vi "Calculate Global Grid Points.vi"(9 "steering frame position":T1, 10 "pictures size (units)":cluster{"width":dbl, "height":dbl}, 11 "grid spacing":dbl=1.0) -> (2 "y":dbl[](array[numeric]), 3 "x":dbl[](array[numeric]))   [LabVIEW 2017, in "NI_Robotics_Configure Steering Frame.lvlib"]
uses:
  <vilib>/robotics/Dialog/Configure Steering Frame/NI_Robotics_Configure Steering Frame.lvlib
  <vilib>/Analysis/coordinate.llb/2D Cartesian Coordinate Shift (Array).vi
  <vilib>/Analysis/coordinate.llb/2D Cartesian Coordinate Rotation (Array).vi
  <vilib>/Analysis/NI_AALPro.lvlib
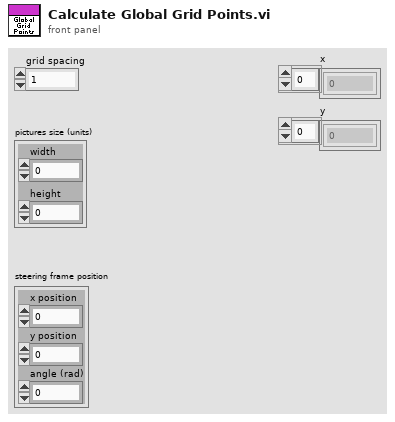
[diagram p1: front panel]
types:
  T1 = cluster{"x position":dbl, "y position":dbl, "angle (rad)":dbl}
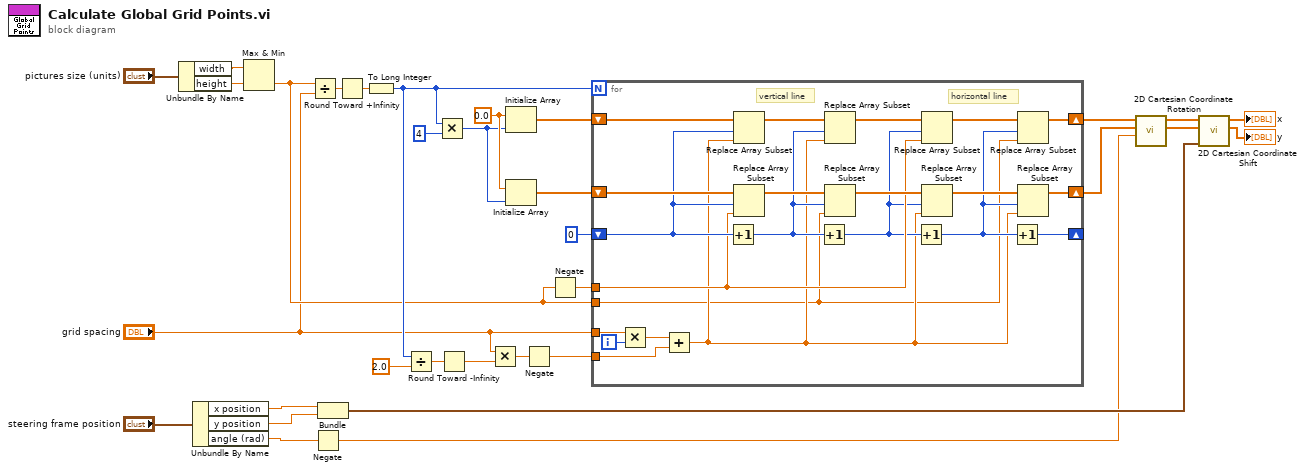
[diagram p0: block diagram]
diagram:
  w26 = 0.0 ("grid spacing")
  n1 = Unbundle By Name("pictures size (units)") -> ("width"=w31:dbl, "height"=w30:dbl)
  n2 = Unbundle By Name("steering frame position") -> ("x position"=w15:dbl, "y position"=w14:dbl, "angle (rad)"=w12:dbl)
  n3 = Max & Min(x=w31, y=w30) -> (min(x,y)=w4:dbl)  [unwired: 1 out]
  n4 = Divide(x=w4, y="grid spacing") -> (x/y=w29:dbl)
  n5 = Negate(x=w12) -> (-x=w11:dbl)
  n6 = Bundle("x position"=w15, "y position"=w14) -> (w13:cluster{"x position":dbl, "y position":dbl})  [unwired: 1 in]
  n7 = Round Toward +Infinity(x=w29) -> (ceil(x): smallest int >= x=w23:dbl)
  n8 = To Long Integer(number=w23) -> (32bit integer=w21:i32)
  n9 = Divide(x=w21, y=2.0) -> (x/y=w20:dbl)
  n10 = Multiply(x=w21, y=4) -> (x*y=w25:i32)
  n11 = Round Toward -Infinity(1:w20) -> (0:w2:dbl)
  n12 = Multiply(x="grid spacing", y=w2) -> (x*y=w1:dbl)
  n13 = Initialize Array(w26, w25) -> (w27:dbl[])
  n14 = Initialize Array(w26, w25) -> (w24:dbl[])
  n15 = Negate(x=w1) -> (-x=w18:dbl)
  n16 = Negate(x=w4) -> (-x=w17:dbl)
  n17 = for {
    N: w21 -> [_]
    shift-right: [w39] -> w10
    shift-left: w27 -> [w50]
    shift-right: [w38] -> w9
    shift-left: w24 -> [w49]
    tunnel: "grid spacing" -> [w54]
    tunnel: w18 -> [w51]
    tunnel: w4 -> [w33]
    shift-right: [w36] -> _
    shift-left: 0 -> [w48]
    tunnel: w17 -> [w42]
    i -> [w53]
    # "horizontal line"
    # "vertical line"
    n18 = Multiply(x=w54, y=w53) -> (x*y=w52:dbl)
    n19 = Add(x=w52, y=w51) -> (x+y=w34:dbl)
    n20 = Increment(x=w48) -> (x+1=w45:i32)
    n21 = Replace Array Subset(array=w50, new element=w34, index=w48) -> (w47:dbl[])
    n22 = Replace Array Subset(array=w49, new element=w42, index=w48) -> (w46:dbl[])
    n23 = Increment(x=w45) -> (x+1=w37:i32)
    n24 = Replace Array Subset(array=w47, new element=w34, index=w45) -> (w44:dbl[])
    n25 = Replace Array Subset(array=w46, new element=w33, index=w45) -> (w43:dbl[])
    n26 = Increment(x=w37) -> (x+1=w35:i32)
    n27 = Replace Array Subset(array=w44, new element=w42, index=w37) -> (w41:dbl[])
    n28 = Replace Array Subset(array=w43, new element=w34, index=w37) -> (w40:dbl[])
    n29 = Increment(x=w35) -> (x+1=w36:i32)
    n30 = Replace Array Subset(array=w41, new element=w33, index=w35) -> (w39:dbl[])
    n31 = Replace Array Subset(array=w40, new element=w34, index=w35) -> (w38:dbl[])
  }
  n32 = call-poly <vilib>:"2D Cartesian Coordinate Rotation.vi"("theta"=w11, "Y"=w9, "X"=w10) -> ("Y Out"=w7:dbl[], "X Out"=w8:dbl[])  [unwired: 6 in, 1 out]
  n33 = call-poly <vilib>:"2D Cartesian Coordinate Shift.vi"("shift"=w13, "Y"=w7, "X"=w8) -> ("Y Out"=→"y":dbl[], "X Out"=→"x":dbl[])  [unwired: 6 in, 1 out]
